vi "TrangeCalc.vi"(7 "error in (no error)":errorcluster) -> (0 "error out":errorcluster, 1 "T2":dbl, 2 "T1":dbl, 3 "array":dbl[](array[numeric]))   [LabVIEW 2019]
uses:
  Durability/common/Global 1.vi
  _ctrl/rw.ctl
panel:
  out "read_dl950":string
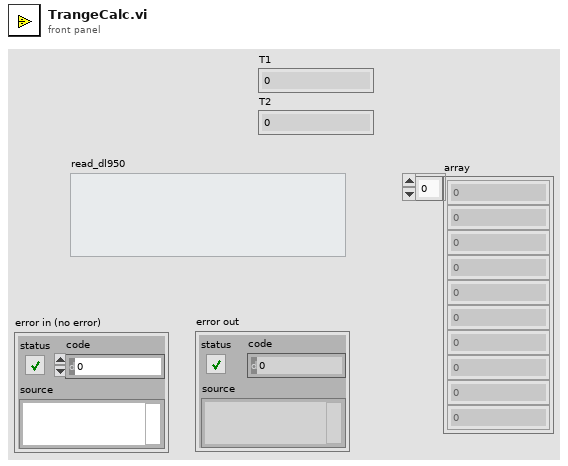
[diagram p1: front panel]
types:
  T1 = typedef "rw.ctl" = enum16{"read", "write"}
  T2 = typedef "Testing-info.ctl" = cluster{"전체채널수":u8, "현재채널번호":u8, "Irms":dbl, "입력전압":dbl, "입력전류":dbl, "출력전압":dbl, "출력전류":dbl, "온도":dbl, "제어단 단선":bool, "제어단 단락":bool, "제어단 특성변화":bool, "출력단 단선":bool, "출력단 단락":bool, "출력단 특성변화":bool, "출력단 전압":bool, "카운트 일치":bool, "Irms 판정":bool, "온도":bool, "테스트 회수":u32, "TestType":T3, "현재회수":u32, "Ch selection":cluster{"1ch":bool, "2ch":bool, "3ch":bool, "4ch":bool, "5ch":bool, "6ch":bool}, "반복":u32, "Path":path, "파일생성주기":u32, "start time":dbl, "stop time":dbl, "현재반복회수":u32, "NG":cluster{"입출력 카운트":bool, "출력전류RMS":bool}}
  T3 = typedef "sequence_single.ctl" = enum16{"Register", "RC", "B1", "B2", "B3", "Oper_LV", "Oper_HV", "ContR_LV"}
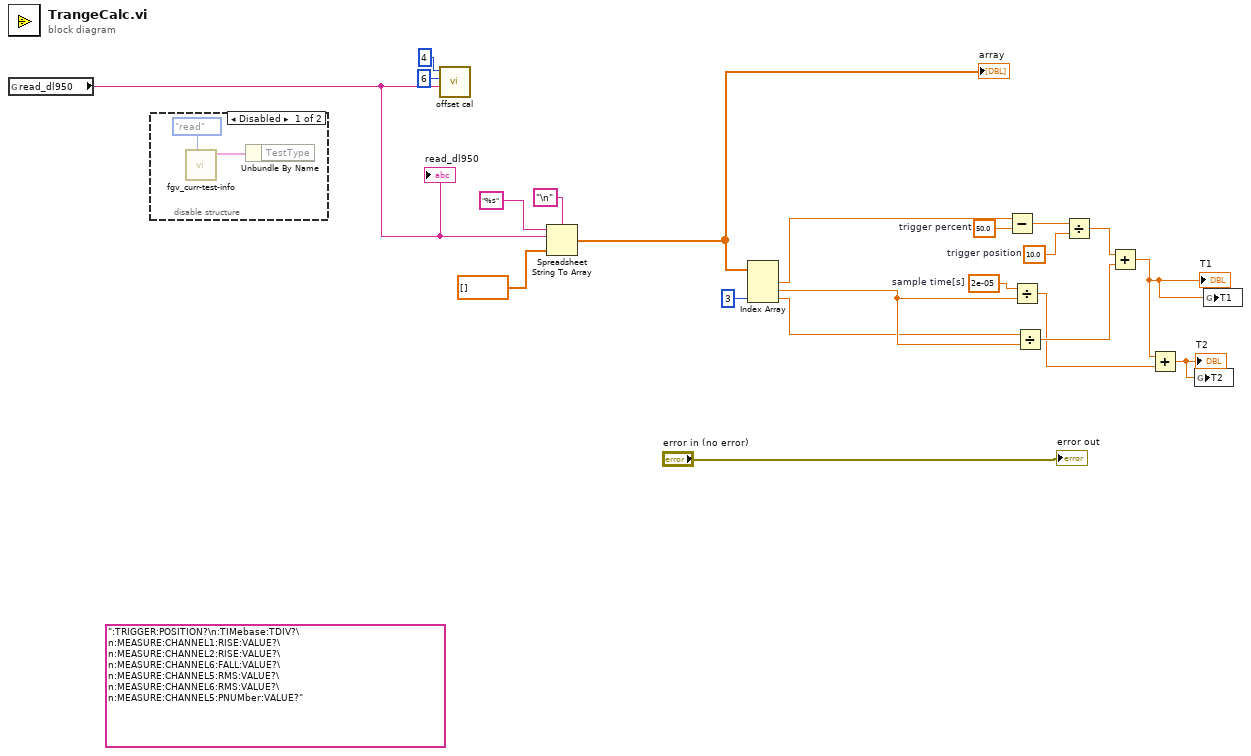
[diagram p0: block diagram]
diagram:
  (unwired) ":TRIGGER:POSITION?\n:TIMebase:TDIV?\n:MEASURE:CHANNEL1:RISE:VALUE?\n:MEASURE:CHANNEL2:RISE:VALUE?\n:MEASURE:CHANNEL6:FALL:VALUE?\n:MEASURE:CHANNEL5:RMS:VALUE?\n:MEASURE:CHANNEL6:RMS:VALUE?\n:MEASURE:CHANNEL5:PNUMber:VALUE?" ("String")
  w8 = 2e-05  # sample time[s]
  w15 = 10.0  # trigger position
  w17 = 50.0  # trigger percent
  n1 = global read "Global 1.vi" "read_dl950"() -> (w4:string)
  "read_dl950" <- w4
  n2 = disable-structure shown="Disabled" {
    frame Disabled {
      n3 = call "fgv_curr-test-info.vi"("cmd"=rw."read") -> ("현재테스트 정보 2"=w22:T2)  [unwired: 10 in]
      n4 = Unbundle By Name(w22) -> ()  [unwired: 1 out]
    }
    frame Enabled {
    }
  }
  n5 = call "offset cal.vi"("read_dl950"=w4, "index low"=6, "index level"=4) -> ()  [unwired: 7 in, 2 out]
  n6 = Spreadsheet String To Array(delimiter (Tab)="\n", format string="%s", spreadsheet string=w4, array type (2D Dbl)=dbl[] []) -> (array=w1:dbl[])
  "array" <- w1
  n7 = Index Array(array=w1, index #3=3 ("index")) -> (element #1=w18:dbl, element #2=w10:dbl, element #3=w9:dbl)  [unwired: 2 in]
  n8 = Subtract(x=w18, y=w17) -> (x-y=w16:dbl)
  n9 = Divide(x=w8, y=w10) -> (x/y=w12:dbl)
  n10 = Divide(x=w9, y=w10) -> (x/y=w13:dbl)
  n11 = Divide(x=w16, y=w15) -> (x/y=w14:dbl)
  n12 = Add(x=w14, y=w13) -> (x+y=w6:dbl)
  "T1" <- w6
  n13 = Add(x=w6, y=w12) -> (x+y=w5:dbl)
  "T2" <- w5
  n14 = global write "Global 1.vi" "T2"(w5) -> ()
  n15 = global write "Global 1.vi" "T1"(w6) -> ()
  "error out" <- "error in (no error)"
